vi "setmotorvelocityonly.vi"(1 "Automation Refnum in":refnum<k7>) -> (0 "motorref out":refnum<k7>)   [LabVIEW 2013]
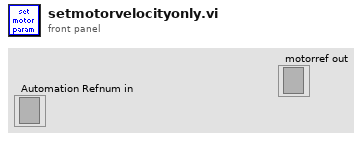
[diagram p1: front panel]
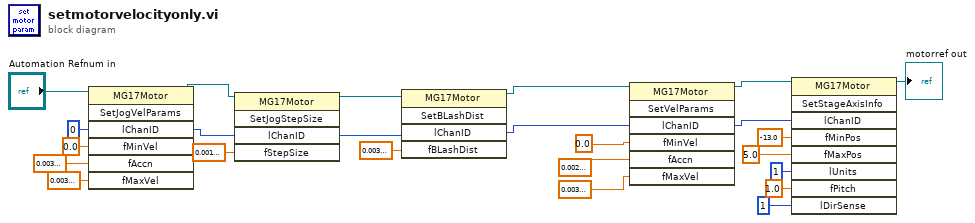
[diagram p0: block diagram]
diagram:
  n1 = invoke class="MG17Motor" method="SetJogVelParams"(reference="Automation Refnum in", "lChanID"=0, "fMinVel"=sgl 0.0, "fAccn"=sgl 0.003, "fMaxVel"=sgl 0.003) -> (reference out=w9:refnum<k7>, "lChanID"=w15:i32)  [unwired: 2 in, 5 out]
  n2 = invoke class="MG17Motor" method="SetJogStepSize"(reference=w9, "lChanID"=w15, "fStepSize"=sgl 0.001) -> (reference out=w12:refnum<k7>, "lChanID"=w16:i32)  [unwired: 2 in, 3 out]
  n3 = invoke class="MG17Motor" method="SetBLashDist"(reference=w12, "lChanID"=w16, "fBLashDist"=sgl 0.003) -> (reference out=w13:refnum<k7>, "lChanID"=w17:i32)  [unwired: 2 in, 3 out]
  n4 = invoke class="MG17Motor" method="SetVelParams"(reference=w13, "lChanID"=w17, "fMinVel"=sgl 0.0, "fAccn"=sgl 0.002, "fMaxVel"=sgl 0.003) -> (reference out=w23:refnum<k7>, "lChanID"=w18:i32)  [unwired: 2 in, 5 out]
  n5 = invoke class="MG17Motor" method="SetStageAxisInfo"(reference=w23, "lChanID"=w18, "fMinPos"=sgl -13.0, "fMaxPos"=sgl 5.0, "lUnits"=1, "fPitch"=sgl 1.0, "lDirSense"=1) -> (reference out=→"motorref out":refnum<k7>)  [unwired: 2 in, 8 out]
